vi "氨氮启动流程.vi"() -> ()   [LabVIEW 2016]
uses:
  <vilib>/Utility/miscctls.llb/LVPointTypeDef.ctl
panel:
  out "空白实测值":sgl
  out "空白数据时间":timestamp
  out "加标回收实测值":sgl
  out "加标回收数据时间":timestamp
  out "跨度核查实测值":sgl
  out "跨度核查数据时间":timestamp
  out "零点核查实测值":sgl
  out "零点核查数据时间":timestamp
  out "水样实测值":sgl
  out "水样数据时间":timestamp
  out "启动记录":string
  out "流程运行中":bool
  out "启动次数":i32
  out "日期/时间":string
  out "运行状态":string
  out "步骤运行时间/秒":i32
  out "流程结束":bool
  out "当前步骤":T1(ring)
  in  "步骤时间/秒":T2={"步骤1时间"=2, "步骤2时间"=4, "步骤3时间"=2, "步骤4时间"=5, "步骤5时间"=6, "步骤6时间"=3, "步骤7时间"=4, "步骤8时间"=7, "步骤9时间"=8, "步骤10时间"=6}
  # "氨氮模块"
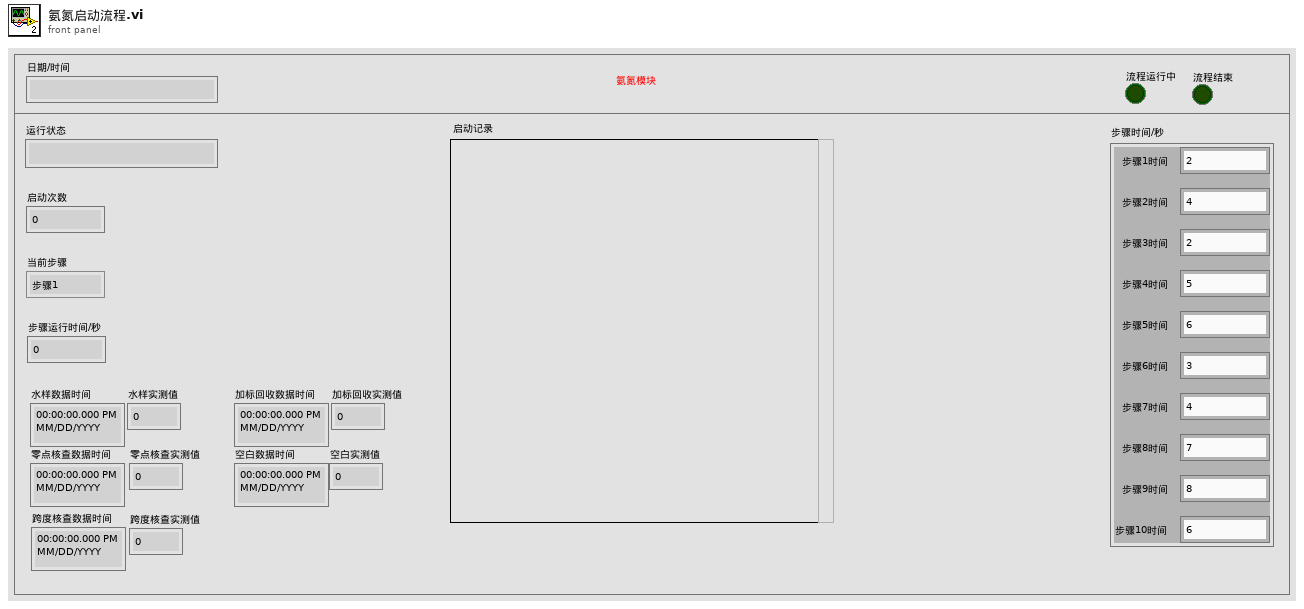
[diagram p1: front panel]
types:
  T1 = enum16{"步骤1", "步骤2", "步骤3", "步骤4", "步骤5", "步骤6", "步骤7", "步骤8", "步骤9", "步骤10"}
  T2 = cluster{"步骤1时间":i32, "步骤2时间":i32, "步骤3时间":i32, "步骤4时间":i32, "步骤5时间":i32, "步骤6时间":i32, "步骤7时间":i32, "步骤8时间":i32, "步骤9时间":i32, "步骤10时间":i32}
  T3 = enum16{"write register", "read register", "write and read register", "write coil", "read coil"}
  T4 = typedef "LVPointTypeDef.ctl" = cluster{"Horizontal":i16, "Vertical":i16}
  T5 = enum32{"Bad", "Idle", "Run top level", "Running"}
  T6 = cluster{"系统时间":timestamp, "工作状态":u16, "测量模式":u16, "告警代码":enum16{"无告警", "缺试剂告警", "缺水样告警", "缺蒸馏水告警", "缺标液告警", "仪表漏液告警", "标定异常告警", "超量程告警", "加热异常", "低试剂预警", "超上限告警", "超下限告警", "仪表内部其他异常", "滴定异常告警", "电极异常告警", "量程切换告警", "参数设置告警", "PH电极电位异常", "电导率电极异常", "浊度光度异常", "溶解氧电极异常", "溶解氧光强异常", "温度异常告警", "PH异常告警", "溶解氧异常告警", "电导率异常告警", "浊度异常告警", "叶绿素异常告警", "藻密度异常告警", "蓝绿藻异常告警", "ORP异常告警", "氨氮异常告警", "清洁刷异常告警", "SD卡异常告警", "蓝牙异常告警", "Wifi异常告警", "流程异常告警"}, "故障代码":enum16{"无故障", "电机故障", "温度故障", "通讯故障", "滴定故障"}, "日志代码":u16, "软件版本":u16, "F0":sgl, "F1":sgl, "F2":sgl, "F3":sgl, "T":sgl, "H":sgl, "id":u16, "flowid":u16, "量程":u16}
  T7 = cluster{"因子编码":u32, "单位":u16, "标样参考值":sgl, "水样数据时间":timestamp, "水样实测值":sgl, "水样数据标识":string, "标样数据时间":timestamp, "标样实测值":sgl, "标样数据标识":string, "空白数据时间":timestamp, "空白实测值":sgl, "空白数据标识":string, "零点核查数据时间":timestamp, "零点核查实测值":sgl, "零点核查数据标识":string, "跨度核查数据时间":timestamp, "跨度核查实测值":sgl, "跨度核查数据标识":string, "加标回收数据时间":timestamp, "加标回收实测值":sgl, "加标回收数据标识":string, "平行样数据时间":timestamp, "平行样实测值":sgl, "平行样数据标识":string}
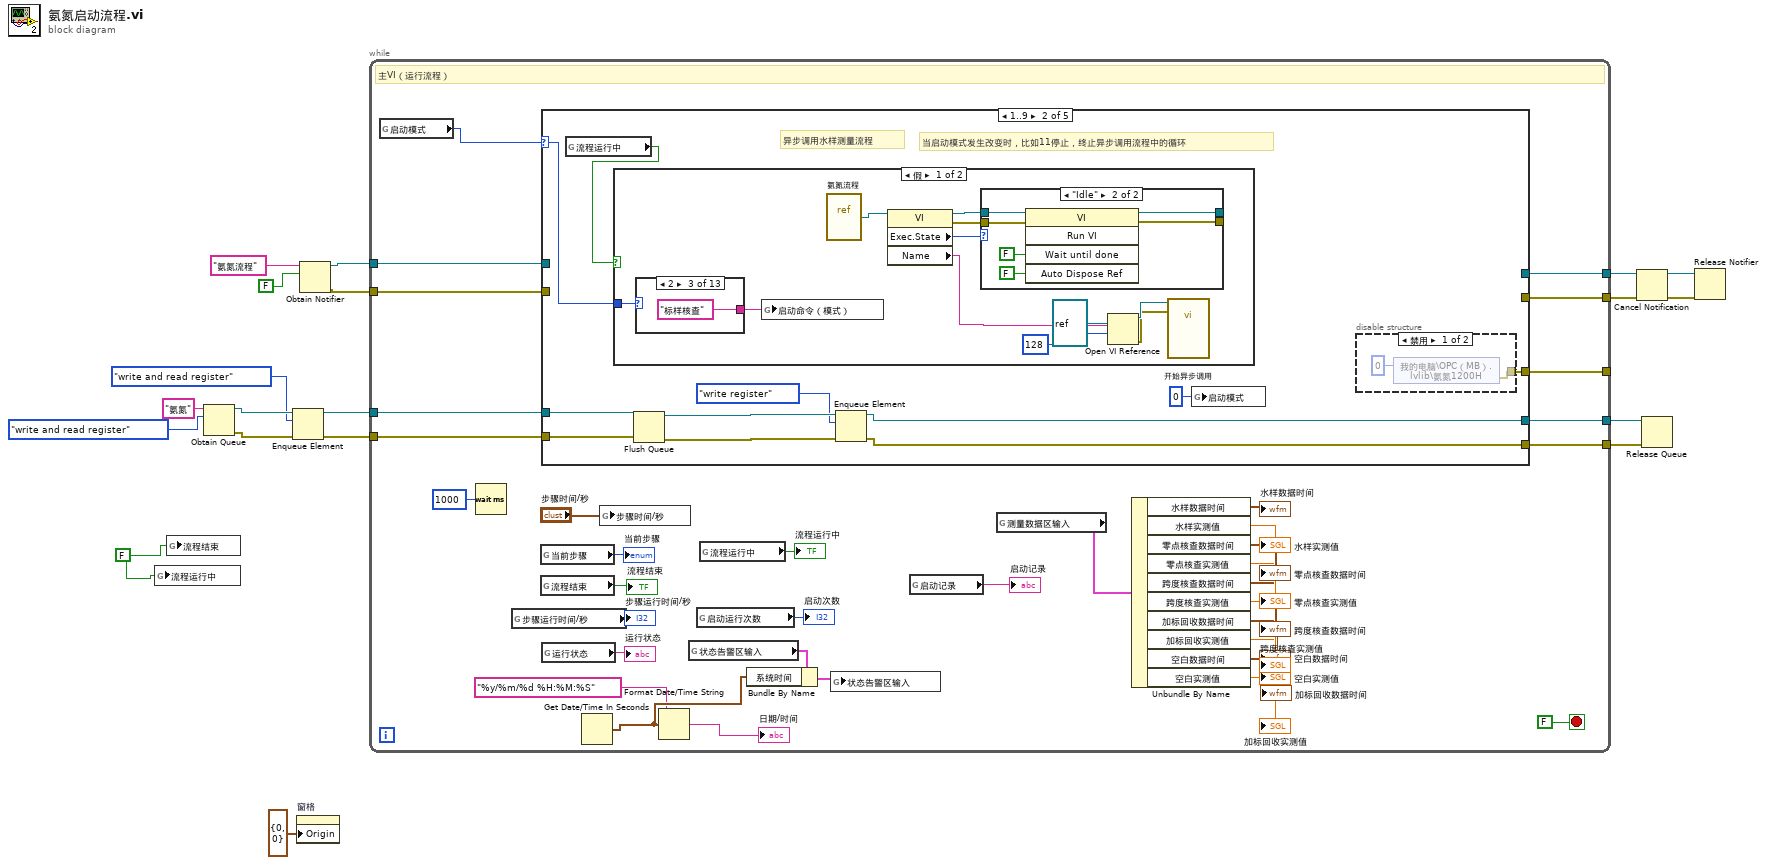
[diagram p0: block diagram]
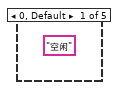
[diagram p2: hidden frame]
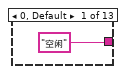
[diagram p4: hidden frame]
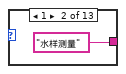
[diagram p5: hidden frame]
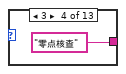
[diagram p6: hidden frame]
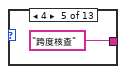
[diagram p7: hidden frame]
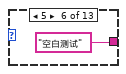
[diagram p8: hidden frame]
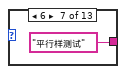
[diagram p9: hidden frame]
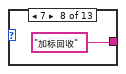
[diagram p10: hidden frame]
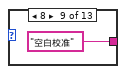
[diagram p11: hidden frame]
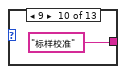
[diagram p12: hidden frame]
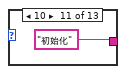
[diagram p13: hidden frame]
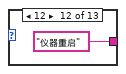
[diagram p14: hidden frame]
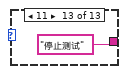
[diagram p15: hidden frame]
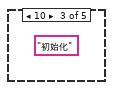
[diagram p18: hidden frame]
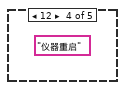
[diagram p19: hidden frame]
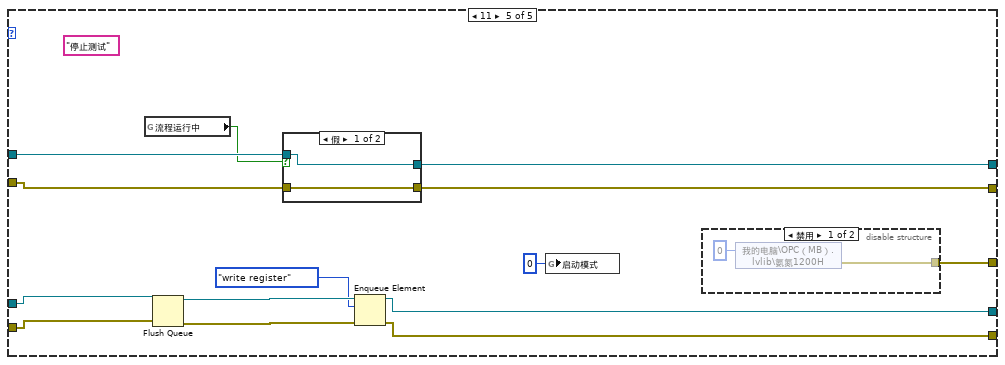
[diagram p20: hidden frame]
diagram:
  w10 = FALSE ("流程结束")
  n1 = global write "氨氮全局.vi" "流程运行中"(w10) -> ()
  n2 = global write "氨氮全局.vi" "流程结束"(w10) -> ()
  n3 = Obtain Queue(name (unnamed)="氨氮" ("名称（未命名）"), element data type=T3."write and read register") -> (queue out=w7:refnum<queue>, error out=w6:errorcluster)  [unwired: 3 in, 1 out]
  n4 = Enqueue Element(queue=w7, element=T3."write and read register", error in (no error)=w6) -> (queue out=w4:refnum<queue>, error out=w3:errorcluster)  [unwired: 1 in, 1 out]
  n5 = property on="窗格" class="Pane"("Origin"=T4 {"Horizontal"=0, "Vertical"=0} ("原点")) -> ()  [unwired: 2 in, 2 out]
  n6 = Obtain Notifier(name (unnamed)="氨氮流程" ("名称（未命名）"), notification data type=FALSE) -> (notifier out=w15:refnum<notifier>, error out=w14:errorcluster)  [unwired: 2 in, 1 out]
  n7 = while {
    tunnel: w14 -> [w53]
    tunnel: w15 -> [w52]
    tunnel: [w51] -> w18
    tunnel: [w50] -> w19
    tunnel: w4 -> [w36]
    tunnel: w3 -> [w35]
    tunnel: [w34] -> w2
    tunnel: [w33] -> w1
    tunnel: [w20] -> _
    stop <- FALSE stop-if-true
    # "主VI（运行流程）"
    n8 = global read "氨氮全局.vi" "启动模式"() -> (w21:u16)
    n9 = Wait (ms)(milliseconds to wait=u32 1000 ("等待时间（毫秒）")) -> ()  [unwired: 1 out]
    n10 = global read "氨氮全局.vi" "步骤运行时间/秒"() -> (→"步骤运行时间/秒":i32)
    n11 = global read "氨氮全局.vi" "当前步骤"() -> (→"当前步骤":T1)
    n12 = global read "氨氮全局.vi" "流程结束"() -> (→"流程结束":bool)
    n13 = case shown="1..9" w21 {
      selector: w21 -> [_ w66 _ _ _]
      tunnel: w53 -> [_ _ _ _ w103]
      tunnel: w52 -> [_ _ _ _ w114]
      tunnel: [_ _ _ _ w113] -> w51
      tunnel: [_ _ _ _ w104] -> w50
      tunnel: w36 -> [_ w62 _ _ w109]
      tunnel: w35 -> [_ w61 _ _ w108]
      tunnel: [_ w60 _ _ w107] -> w34
      tunnel: [_ w59 _ _ w106] -> w33
      tunnel: [_ w56 _ _ w101] -> w20
      frame 0, Default {
        (unwired) "空闲"
      }
      frame 1..9 {
        # "当启动模式发生改变时，比如11停止，终止异步调用流程中的循环"
        # "异步调用水样测量流程"
        n14 = global read "氨氮全局.vi" "流程运行中"() -> (w58:bool)
        n15 = case shown="假" w58 {
          tunnel: w66 -> [w70 _]
          frame False {
            n16 = case shown="2" w70 {
              tunnel: ["空闲" "水样测量" "标样核查" "零点核查" "跨度核查" "空白测试" "平行样测试" "加标回收" "空白校准" "标样校准" "初始化" "仪器重启" "停止测试"] -> w69
              frame 0, Default {
              }
              frame 1 {
              }
              frame 2 {
              }
              frame 3 {
              }
              frame 4 {
              }
              frame 5 {
              }
              frame 6 {
              }
              frame 7 {
              }
              frame 8 {
              }
              frame 9 {
              }
              frame 10 {
              }
              frame 12 {
              }
              frame 11 {
              }
            }
            n17 = global write "氨氮全局.vi" "启动命令（模式）"(w69) -> ()
            n18 = vi-ref "氨氮流程.vi"() -> (w79:refnum<vi>)
            n19 = property class="VI"(reference=w79) -> (reference out=w78:refnum<vi>, error out=w76:errorcluster, "Exec.State"=w77:T5, "Name"=w71:string)  [unwired: 1 in]
            n20 = case shown="\"Idle\"" w77 {
              tunnel: w78 -> [w94 w100]
              tunnel: [w94 w99] -> _
              tunnel: w76 -> [w93 w96]
              tunnel: [w93 w95] -> _
              frame "Bad", Default {
              }
              frame "Idle" {
                n21 = invoke class="VI" method="Run VI"(reference=w100, error in=w96, "Wait until done"=FALSE ("结束前等待"), "Auto Dispose Ref"=FALSE ("自动销毁引用")) -> (reference out=w99:refnum<vi>, error out=w95:errorcluster)  [unwired: 1 in, 3 out]
              }
            }
            n22 = Open VI Reference(type specifier VI Refnum (for type only)=refnum<vi> refnum ("类型说明符VI引用句柄（仅用于类型）"), vi path=w71, options=128 ("选项")) -> (vi reference=w75:refnum<vi>, error out=w73:errorcluster)  [unwired: 3 in]
            n23 = call-by-ref "开始异步调用"(reference=w75, error in=w73) -> ()  [unwired: 12 in, 2 out]
          }
          frame True {
          }
        }
        n24 = Flush Queue(queue=w62, error in (no error)=w61) -> (queue out=w65:refnum<queue>, error out=w64:errorcluster)  [unwired: 1 out]
        n25 = Enqueue Element(queue=w65, element=T3."write register", error in (no error)=w64) -> (queue out=w60:refnum<queue>, error out=w59:errorcluster)  [unwired: 1 in, 1 out]
        n26 = global write "氨氮全局.vi" "启动模式"(u16 0 ("启动模式")) -> ()
        n27 = disable-structure shown="禁用" {
          disable-tunnel: [w68 _] -> w56
          frame Disabled {
            n28 = shared-variable "我的电脑\\OPC（MB）.lvlib\\氨氮1200H"(u16 0 ("氨氮1200H")) -> (error out=w68:errorcluster)  [unwired: 1 in]
          }
          frame Enabled {
          }
        }
      }
      frame 10 {
        (unwired) "初始化"
      }
      frame 12 {
        (unwired) "仪器重启"
      }
      frame 11 {
        (unwired) "停止测试"
        n29 = global read "氨氮全局.vi" "流程运行中"() -> (w105:bool)
        n30 = Flush Queue(queue=w109, error in (no error)=w108) -> (queue out=w112:refnum<queue>, error out=w111:errorcluster)  [unwired: 1 out]
        n31 = case shown="假" w105 {
          tunnel: w114 -> [w118 w122]
          tunnel: [w118 w121] -> w113
          tunnel: [w117 w120] -> w104
          tunnel: w103 -> [w117 w119]
          frame False {
          }
          frame True {
            n32 = Send Notification(notification=TRUE ("通知"), notifier=w122, error in (no error)=w119) -> (notifier out=w121:refnum<notifier>, error out=w120:errorcluster)
          }
        }
        n33 = Enqueue Element(queue=w112, element=T3."write register", error in (no error)=w111) -> (queue out=w107:refnum<queue>, error out=w106:errorcluster)  [unwired: 1 in, 1 out]
        n34 = global write "氨氮全局.vi" "启动模式"(u16 0 ("启动模式")) -> ()
        n35 = disable-structure shown="禁用" {
          disable-tunnel: [w115 _] -> w101
          frame Disabled {
            n36 = shared-variable "我的电脑\\OPC（MB）.lvlib\\氨氮1200H"(u16 0 ("氨氮1200H")) -> (error out=w115:errorcluster)  [unwired: 1 in]
          }
          frame Enabled {
          }
        }
      }
    }
    n37 = global read "氨氮全局.vi" "运行状态"() -> (→"运行状态":string)
    n38 = Get Date/Time In Seconds() -> (seconds since 1Jan1904=w47:timestamp)
    n39 = global write "氨氮全局.vi" "步骤时间/秒"("步骤时间/秒") -> ()
    n40 = Format Date/Time String(time format string (%c)="%y/%m/%d %H:%M:%S" ("时间格式字符串(%c)"), seconds (now)=w47) -> (date/time string=→"日期/时间":string)  [unwired: 1 in]
    n41 = global read "氨氮全局.vi" "状态告警区输入"() -> (w45:T6)
    n42 = global read "氨氮全局.vi" "启动运行次数"() -> (→"启动次数":i32)
    n43 = global read "氨氮全局.vi" "流程运行中"() -> (→"流程运行中":bool)
    n44 = Bundle By Name(cluster=w45, "系统时间"=w47) -> (w46:T6)
    n45 = global write "氨氮全局.vi" "状态告警区输入"(w46) -> ()
    n46 = global read "氨氮全局.vi" "启动记录"() -> (→"启动记录":string)
    n47 = global read "氨氮全局.vi" "测量数据区输入"() -> (w32:T7)
    n48 = Unbundle By Name(w32) -> ("水样数据时间"=→"水样数据时间":timestamp, "水样实测值"=→"水样实测值":sgl, "零点核查数据时间"=→"零点核查数据时间":timestamp, "零点核查实测值"=→"零点核查实测值":sgl, "跨度核查数据时间"=→"跨度核查数据时间":timestamp, "跨度核查实测值"=→"跨度核查实测值":sgl, "加标回收数据时间"=→"加标回收数据时间":timestamp, "加标回收实测值"=→"加标回收实测值":sgl, "空白数据时间"=→"空白数据时间":timestamp, "空白实测值"=→"空白实测值":sgl)
  }
  n49 = Cancel Notification(0:w18, 3:w19) -> (8:w17:refnum<notifier>, 11:w16:errorcluster)  [unwired: 1 out]
  n50 = Release Queue(queue=w2, error in (no error)=w1) -> ()  [unwired: 1 in, 3 out]
  n51 = Release Notifier(notifier=w17, error in (no error)=w16) -> ()  [unwired: 1 in, 3 out]
